vi "sentinel_emailer.vi"() -> ()   [LabVIEW 2011]
panel:
  in  "Email Alert - CC":string
  in  "Email ALert - Attachment":path
  in  "Email Alert - Message":string="An alarm event has ocurred on a semiconductor test lot that you have requested to monitor.  Please see the attached data log for event details.\n\nThis message is generated automatically by the Sentinel Controller program.\n\nTo stop these messages, please contact the test floor operator and disable automatic alert notifictions.\n\n"
  in  "Email Alert - Engineer":string
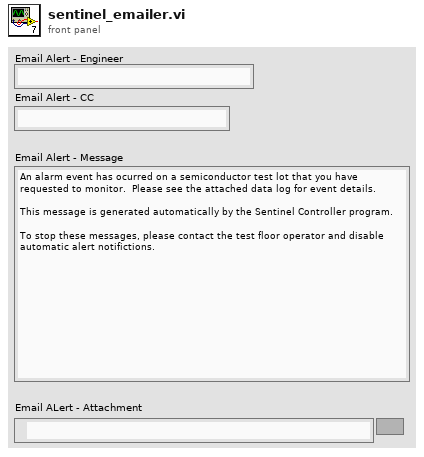
[diagram p1: front panel]
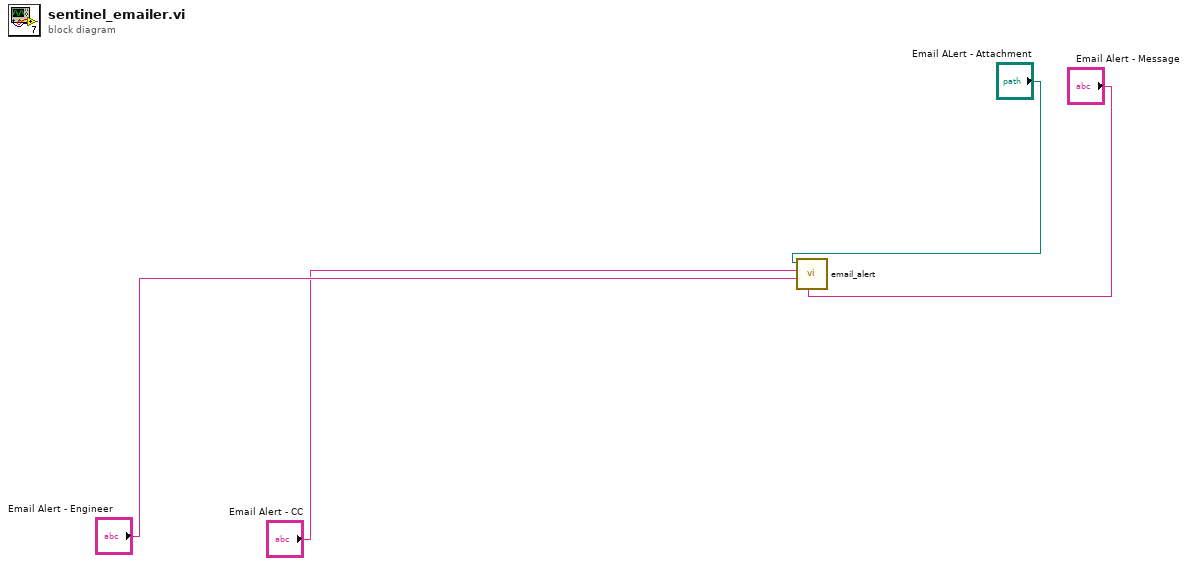
[diagram p0: block diagram]
diagram:
  n1 = call "email_alert.vi"("Email Alert - Message"="Email Alert - Message", "Email Alert - Engineer"="Email Alert - Engineer", "Email Alert - CC"="Email Alert - CC", "Email ALert - Attachment"="Email ALert - Attachment") -> ()  [unwired: 8 in]
